vi "RDS Serial Handler Initialize.vi"(7 "Termination Char(s)":string, 8 "error in (no error)":errorcluster, 9 "baud rate (9600)":u32=9600, 10 "VISA resource name":refnum<visa-resource-name>="COM1", 11 "RDS Serial Instrument in":refnum<class "RDS Serial Instrument.lvclass">) -> (0 "error out":errorcluster, 3 "RDS Serial Instrument out":refnum<class "RDS Serial Instrument.lvclass">)   [LabVIEW 2015, in "RDS Serial Handler.lvlib" / "RDS Serial Instrument.lvclass"]
uses:
  RDS Serial Instrument.lvclass
  RDS Serial Instrument.lvclass/RDS Serial Instrument.ctl
  <vilib>/Instr/_visa.llb/VISA Configure Serial Port (Instr).vi
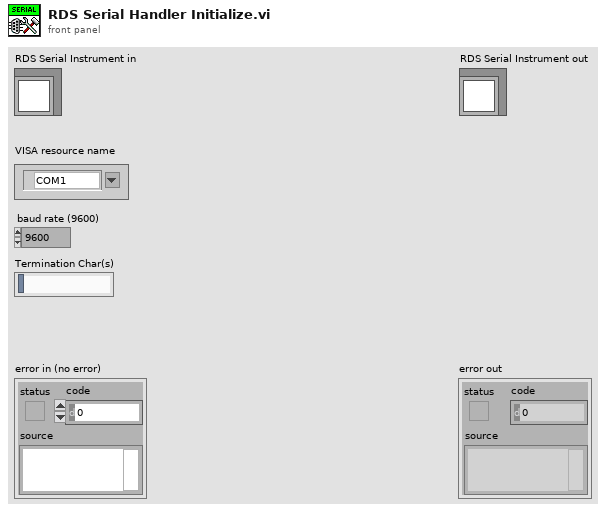
[diagram p1: front panel]
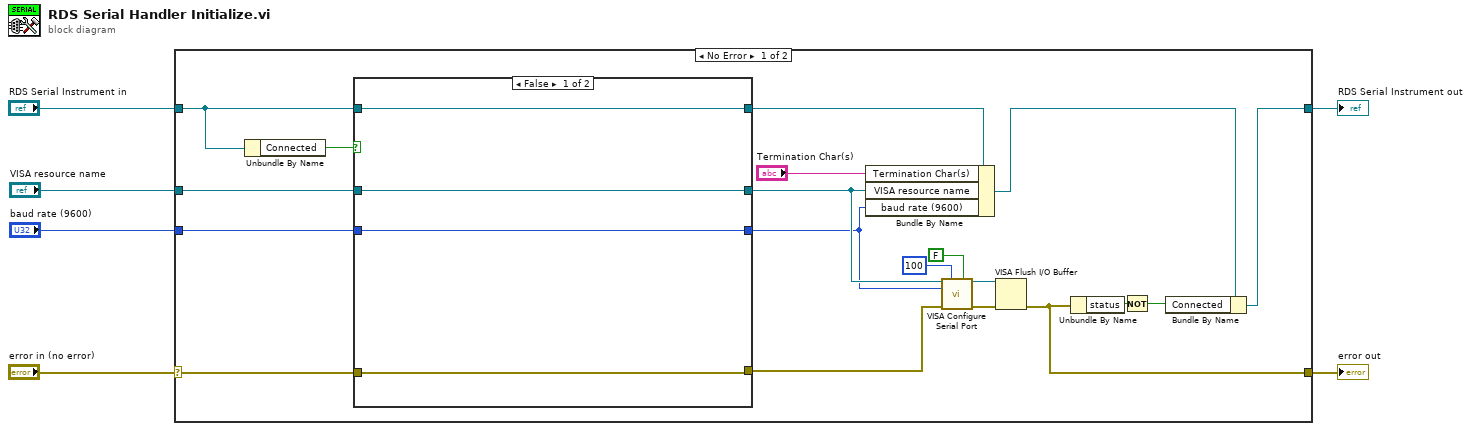
[diagram p0: block diagram]
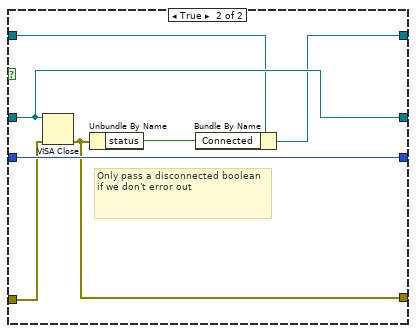
[diagram p2: hidden frame]
diagram:
  n1 = case shown="No Error" "error in (no error)" {
    selector: "error in (no error)" -> [w17 w38]
    tunnel: [w7 w38] -> w5
    tunnel: [w14 w37] -> w3
    tunnel: "RDS Serial Instrument in" -> [w19 w37]
    tunnel: "VISA resource name" -> [w22 _]
    tunnel: "baud rate (9600)" -> [w21 _]
    frame No Error {
      n2 = Unbundle By Name(w19) -> ("Connected"=w18:bool)
      n3 = case shown="False" w18 {
        tunnel: [w27 w32] -> w24
        tunnel: w19 -> [w27 w33]
        tunnel: [w29 w34] -> w23
        tunnel: w22 -> [w29 w34]
        tunnel: w21 -> [w28 w36]
        tunnel: [w28 w36] -> w20
        tunnel: w17 -> [w26 w35]
        tunnel: [w26 w31] -> w16
        frame False {
        }
        frame True {
          # "Only pass a disconnected boolean if we don't error out"
          n4 = VISA Close(VISA resource name=w34, error in (no error)=w35) -> (error out=w31:errorcluster)
          n5 = Unbundle By Name(w31) -> ("status"=w30:bool)
          n6 = Bundle By Name(cluster=w33, "Connected"=w30) -> (w32:refnum<class "RDS Serial Instrument.lvclass">)
        }
      }
      n7 = Bundle By Name(cluster=w24, "Termination Char(s)"="Termination Char(s)", "VISA resource name"=w23, "baud rate (9600)"=w20) -> (w15:refnum<class "RDS Serial Instrument.lvclass">)
      n8 = call-poly "VISA Configure Serial Port"("VISA resource name"=w23, "timeout (10sec)"=u32 100, "Enable Termination\nChar (T)"=FALSE ("Enable Termination\nChar (T)"), "baud rate (9600)"=w20, "error in (no error)"=w16) -> ("VISA resource name out"=w9:refnum<visa-resource-name>, "error out"=w8:errorcluster)  [unwired: 5 in, 4 out]
      n9 = VISA Flush I/O Buffer(VISA resource name=w9, error in (no error)=w8) -> (error out=w7:errorcluster)  [unwired: 1 in, 1 out]
      n10 = Unbundle By Name(w7) -> ("status"=w12:bool)
      n11 = Not(x=w12) -> (.not. x?=w13:bool)
      n12 = Bundle By Name(cluster=w15, "Connected"=w13) -> (w14:refnum<class "RDS Serial Instrument.lvclass">)
    }
    frame Error {
    }
  }
  "error out" <- w5
  "RDS Serial Instrument out" <- w3
